vi "Profile_MaxMinDiffOverMean.vi"() -> (0 "New Values In":string[][](array[string])=[["Test data5"]], 1 "New Chs In":string[](array[string])=["30-10-03:New:Channel new5"])   [LabVIEW 2021]
uses:
  Results_plotter_Global.vi
  <vilib>/Analysis/NI_AALBase.lvlib
  <vilib>/Analysis/baseanly.llb/Mean (DBL).vi
  Data plotting/subVIs/Plot_Values_Global.vi
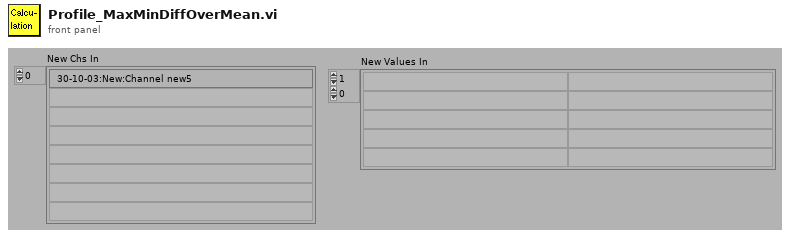
[diagram p1: front panel]
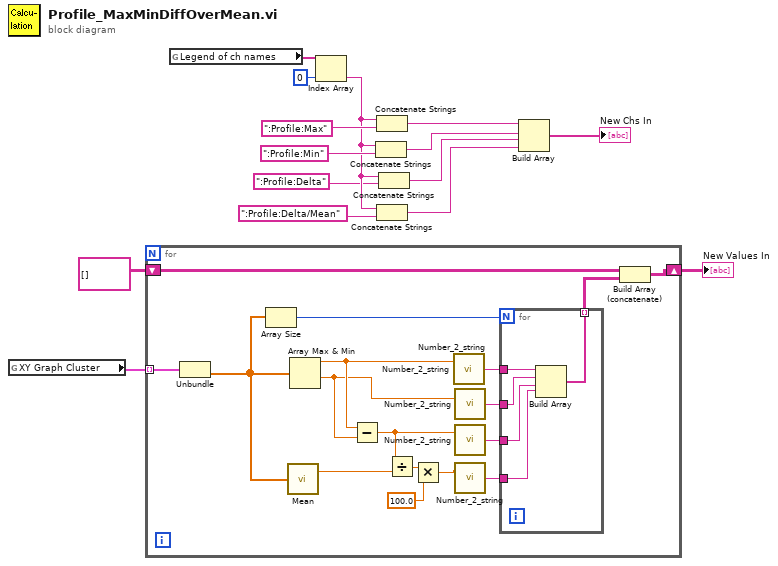
[diagram p0: block diagram]
diagram:
  n1 = global read "Plot_Values_Global.vi" "XY Graph Cluster"() -> (w1:cluster{dbl[], dbl[]}[])
  n2 = for {
    tunnel: w1 -> [w32] mode=indexing
    shift-right: [w30] -> w11
    shift-left: string[][] [] -> [w31]
    n3 = Unbundle(w32) -> (w23:dbl[])  [unwired: 1 out]
    n4 = Array Size(array=w23) -> (size(s)=w28:i32)
    n5 = call-poly <vilib>:"Mean.vi"("X"=w23) -> ("mean"=w21:dbl)  [unwired: 1 out]
    n6 = Array Max & Min(array=w23) -> (max value=w25:dbl, min value=w24:dbl)  [unwired: 2 out]
    n7 = Subtract(x=w25, y=w24) -> (x-y=w22:dbl)
    n8 = Divide(x=w22, y=w21) -> (x/y=w19:dbl)
    n9 = Multiply(x=w19, y=100.0) -> (x*y=w17:dbl)
    n10 = call "Number_2_string.vi"() -> ()  [unwired: 2 in, 1 out]
    n11 = call "Number_2_string.vi"("number"=w25) -> ("String"=w29:string)  [unwired: 1 in]
    n12 = call "Number_2_string.vi"("number"=w24) -> ("String"=w26:string)  [unwired: 1 in]
    n13 = call "Number_2_string.vi"("number"=w22) -> ("String"=w20:string)  [unwired: 1 in]
    n14 = call "Number_2_string.vi"("number"=w17) -> ("String"=w16:string)  [unwired: 1 in]
    n15 = for {
      N: w28 -> [_]
      tunnel: w29 -> [w37]
      tunnel: [w36] -> w27 mode=indexing
      tunnel: w26 -> [w35]
      tunnel: w20 -> [w34]
      tunnel: w16 -> [w33]
      n16 = Build Array(w37, w35, w34, w33) -> (w36:string[])
    }
    n17 = Build Array (concatenate)(w31, w27) -> (w30:string[][])
  }
  "New Values In" <- w11
  n18 = global read "Results_plotter_Global.vi" "Legend of ch names"() -> (w13:string[])
  n19 = Index Array(array=w13, index=0) -> (element=w3:string)
  n20 = Concatenate Strings(w3, ":Profile:Min" ("string")) -> (w6:string)
  n21 = Concatenate Strings(w3, ":Profile:Max" ("string")) -> (w9:string)
  n22 = Concatenate Strings(w3, ":Profile:Delta/Mean" ("string")) -> (w4:string)
  n23 = Concatenate Strings(w3, ":Profile:Delta" ("string")) -> (w5:string)
  n24 = Build Array(w9, w6, w5, w4) -> (→"New Chs In":string[])
